vi "MIMIC Port Close.vi"(1 "VISA resource name":refnum<visa-resource-name>) -> (0 "error out":errorcluster)   [LabVIEW 2014]
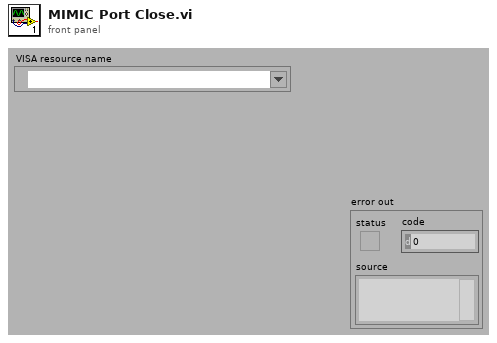
[diagram p1: front panel]
types:
  T1 = enum16{"Initial Serial Port", "Write", "Read", "Close", "ClearBuff"}
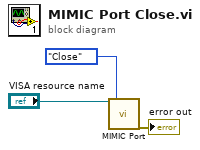
[diagram p0: block diagram]
diagram:
  n1 = call "MIMIC Port.vi"("VISA resource name"="VISA resource name", "Function"=T1."Close") -> ("error out"=→"error out":errorcluster)  [unwired: 14 in, 3 out]
